vi "allocate functions.vi"() -> (1 "functions":T1[](array[typedef]), 2 "instance identifier":string, 3 "tag bus processing plugin module configuration out":refnum<class "Logic Sequencer configuration.lvclass">)   [LabVIEW 2013, in "Logic Sequencer tests.lvlib"]
uses:
  Logic Sequencer tests.lvlib
  module/configuration/processing channels.ctl
  <vilib>/NI/Tag Bus Module Framework/channel/TBM channel.lvclass
  module/configuration/Logic Sequencer configuration.lvclass
  <vilib>/NI/Tag Bus Module Framework/root configuration/TBM configuration.lvclass/TBM configuration.ctl
  <vilib>/NI/Tag Bus Module Framework/channel/channel classification.ctl
  <vilib>/NI/Tag Bus Module Framework/root configuration/Read instance name.vi
  <vilib>/NI/Tag Bus Module Framework/root configuration/TBM configuration.lvclass
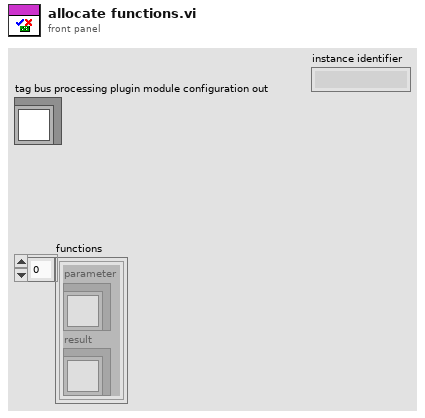
[diagram p1: front panel]
types:
  T1 = typedef "Logic Sequencer configuration.lvclass/processing channels.ctl" = cluster{"parameter":refnum<class "TBM channel.lvclass">, "result":refnum<class "TBM channel.lvclass">}
  T2 = typedef "tag bus.lvlib/tag descriptor.lvclass/Data Type.ctl" = enum16{"Double", "Single", "I64", "I32", "I16", "I8", "U64", "U32", "U16", "U8", "Boolean", "String", "Array of Double", "Array of Single", "Array of I64", "Array of I32", "Array of I16", "Array of I8", "Array of U64", "Array of U32", "Array of U16", "Array of U8", "Array of Boolean", "Array of String"}
  T3 = typedef "TBM channel.lvclass/channel classification.ctl" = enum16{"input data", "output data", "processing parameter", "processing result"}
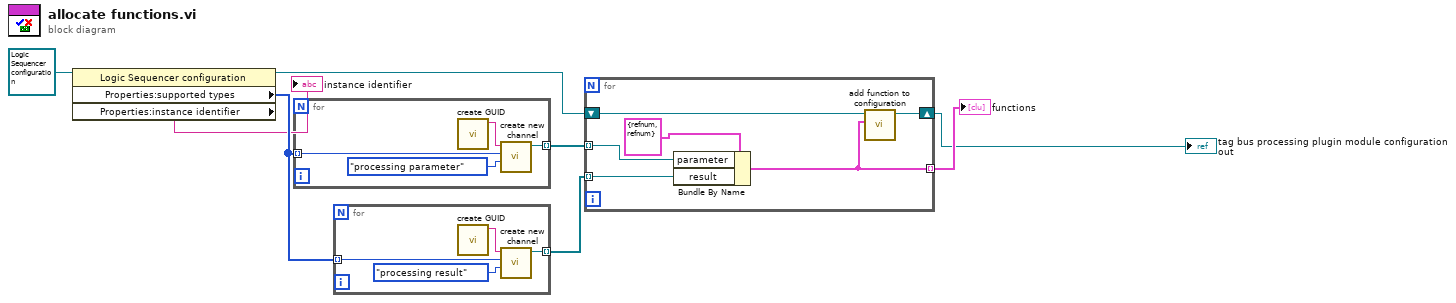
[diagram p0: block diagram]
diagram:
  n1 = property class="Logic Sequencer configuration"(reference=refnum<class "Logic Sequencer configuration.lvclass"> refnum ("tag bus configurable plugin module configuration")) -> (reference out=w2:refnum<class "Logic Sequencer configuration.lvclass">, "Properties:supported types"=w5:T2[], "Properties:instance identifier"=→"instance identifier":string)  [unwired: 1 in, 1 out]
  n2 = for {
    tunnel: [w12] -> w6 mode=indexing
    tunnel: w5 -> [w11] mode=indexing
    n3 = call <vilib>:"create GUID.vi"() -> ("uuid"=w10:string)  [unwired: 11 in]
    n4 = call <vilib>:"create new channel.vi"("channel classification"=channel_classification."processing parameter", "data type"=w11, "channel name"=w10) -> ("channel"=w12:refnum<class "TBM channel.lvclass">)  [unwired: 8 in]
  }
  n5 = for {
    tunnel: [w16] -> w7 mode=indexing
    tunnel: w5 -> [w15] mode=indexing
    n6 = call <vilib>:"create GUID.vi"() -> ("uuid"=w14:string)  [unwired: 11 in]
    n7 = call <vilib>:"create new channel.vi"("channel classification"=channel_classification."processing result", "data type"=w15, "channel name"=w14) -> ("channel"=w16:refnum<class "TBM channel.lvclass">)  [unwired: 8 in]
  }
  n8 = for {
    tunnel: w6 -> [w21] mode=indexing
    tunnel: w7 -> [w20] mode=indexing
    tunnel: [w17] -> w8 mode=indexing
    shift-right: [w18] -> w1
    shift-left: w2 -> [w19]
    n9 = Bundle By Name(cluster=T1 {"parameter"=refnum, "result"=refnum} ("processing cluster"), "parameter"=w21, "result"=w20) -> (w17:T1)
    n10 = call "add function to configuration.vi"("processing function"=w17, "Logic Sequencer configuration in"=w19) -> ("Logic Sequencer configuration out"=w18:refnum<class "Logic Sequencer configuration.lvclass">)  [unwired: 8 in, 1 out]
  }
  "functions" <- w8
  "tag bus processing plugin module configuration out" <- w1
